vi "CheckStepNameLengthAnalysisModule.vi"(0 "AnalysisContext":refnum<k7>) -> (1 "status":bool, 2 "code":i32, 3 "source":string)   [LabVIEW 2011]
uses:
  StepNameLengthRuleConstants.vi
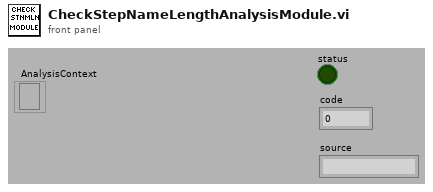
[diagram p1: front panel]
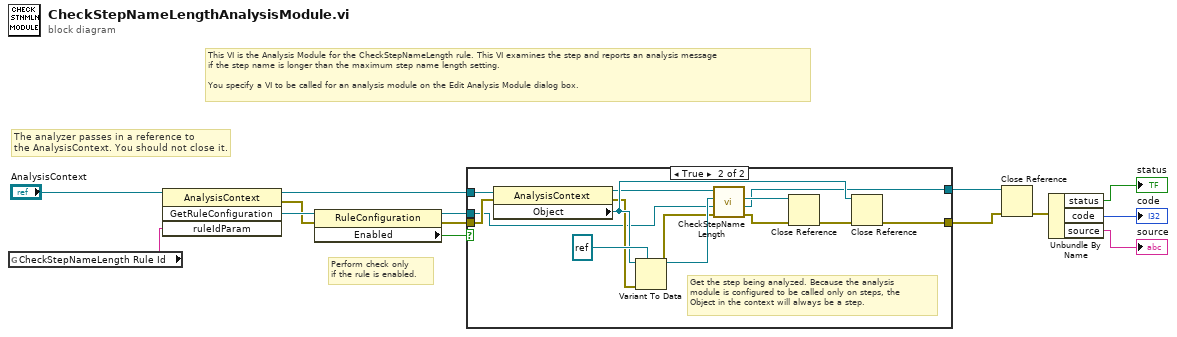
[diagram p0: block diagram]
diagram:
  # "Perform check only\nif the rule is enabled."
  # "The analyzer passes in a reference to\nthe AnalysisContext. You should not close it."
  # "This VI is the Analysis Module for the CheckStepNameLength rule. This VI examines the step and reports an analysis message\nif the step name is longer than the maximum step name length setting.\n\nYou specify a VI to be called for an analysis module on the Edit Analysis Module dialog box."
  n1 = global read "StepNameLengthRuleConstants.vi" "CheckStepNameLength Rule Id"() -> (w9:string)
  n2 = invoke class="AnalysisContext" method="GetRuleConfiguration"(reference="AnalysisContext", "ruleIdParam"=w9) -> (reference out=w10:refnum<k7>, error out=w12:errorcluster, "GetRuleConfiguration"=w13:refnum<k7>)  [unwired: 2 in, 1 out]
  n3 = property class="RuleConfiguration"(reference=w13, error in=w12) -> (reference out=w6:refnum<k7>, error out=w5:errorcluster, "Enabled"=w7:bool)
  n4 = case shown="True" w7 {
    tunnel: w6 -> [w16 w22]
    tunnel: [w16 w19] -> w11
    tunnel: w5 -> [w15 w29]
    tunnel: [w15 w27] -> w8
    tunnel: w10 -> [_ w30]
    frame False {
    }
    frame True {
      # "Get the step being analyzed. Because the analysis\nmodule is configured to be called only on steps, the\nObject in the context will always be a step."
      n5 = property class="AnalysisContext"(reference=w30, error in=w29) -> (reference out=w23:refnum<k7>, error out=w25:errorcluster, "Object"=w26:refnum<k7>)
      n6 = Variant To Data(error in=w25, type=refnum<k7> refnum ("TS.Step"), Variant=w26) -> (data=w24:refnum<k7>, error out=w21:errorcluster)
      n7 = call "CheckStepNameLength.vi"("error in (no error)"=w21, "RuleConfiguration In"=w22, "Step In"=w24, "AnalysisContext In"=w23) -> ("error out"=w18:errorcluster, "RuleConfiguration Out"=w19:refnum<k7>, "Step Out"=w20:refnum<k7>)  [unwired: 5 out]
      n8 = Close Reference(reference=w20, error in (no error)=w18) -> (error out=w17:errorcluster)
      n9 = Close Reference(reference=w26, error in (no error)=w17) -> (error out=w27:errorcluster)
    }
  }
  n10 = Close Reference(reference=w11, error in (no error)=w8) -> (error out=w4:errorcluster)
  n11 = Unbundle By Name(w4) -> ("status"=→"status":bool, "code"=→"code":i32, "source"=→"source":string)
